vi "RT_Test_RS232.vi"() -> ()   [LabVIEW 2018]
uses:
  ControlLoop/TurboPump/Ctl/Function_of_TC110.ctl
panel:
  out "output cluster":T1
  in  "error in (no error)":errorcluster
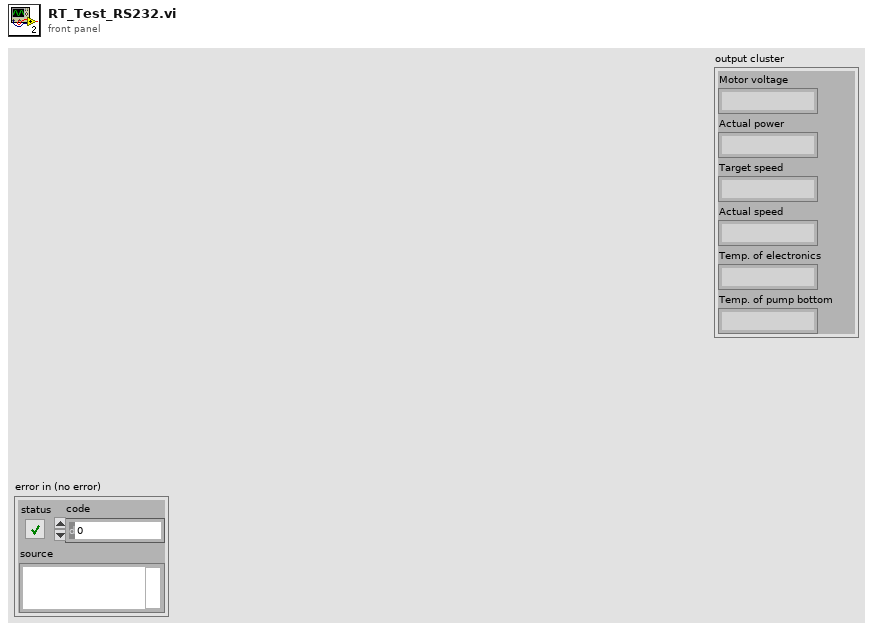
[diagram p1: front panel]
types:
  T1 = cluster{"Motor voltage":string, "Actual power":string, "Target speed":string, "Actual speed":string, "Temp. of electronics":string, "Temp. of pump bottom":string}
  T2 = typedef "Function_of_TC110.ctl" = enum16{"Initialisation", "Read status", "Write command", "Read command"}
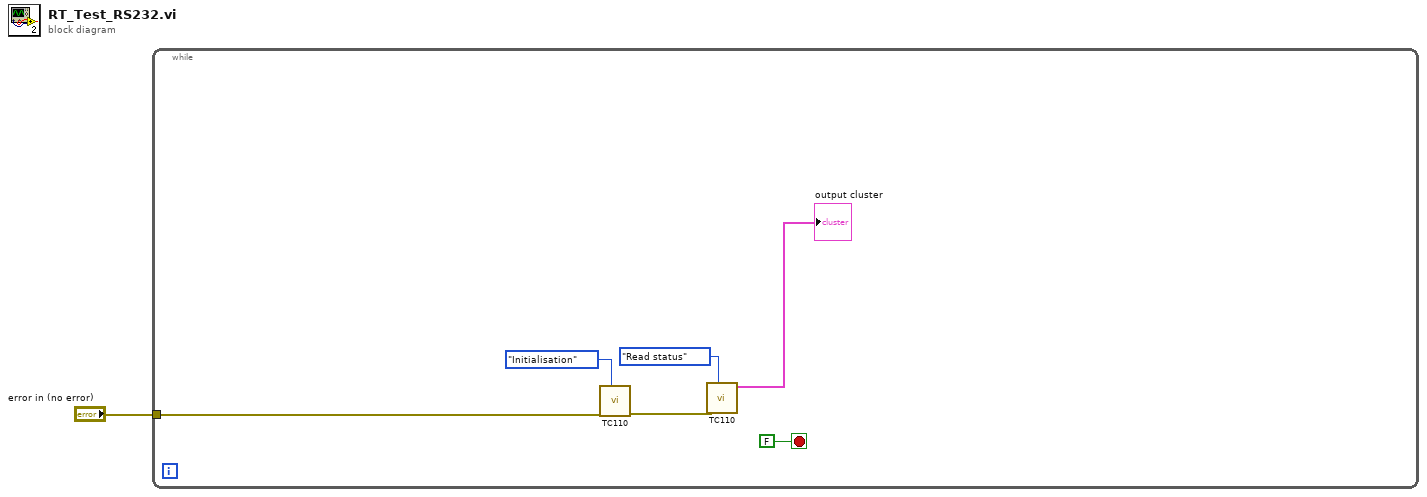
[diagram p0: block diagram]
diagram:
  n1 = while {
    tunnel: "error in (no error)" -> [w4]
    stop <- FALSE stop-if-true
    n2 = call "TC110.vi"("Function"=Function_of_TC110."Initialisation", "Error in"=w4) -> ("Error out"=w5:errorcluster)  [unwired: 6 in, 3 out]
    n3 = call "TC110.vi"("Function"=Function_of_TC110."Read status", "Error in"=w5) -> ("output cluster"=→"output cluster":T1)  [unwired: 6 in, 3 out]
  }
